vi "Read_Bid.vi"(8 "error in (no error)":errorcluster, 11 "Modbus master in":refnum<class "Modbus Master.lvclass">) -> (0 "error out":errorcluster, 2 "Variables":sgl[](array[numeric]), 3 "Modbus master out":refnum<class "Modbus Master.lvclass">)   [LabVIEW 2017]
uses:
  <vilib>/Modbus/master/Modbus Master.lvclass
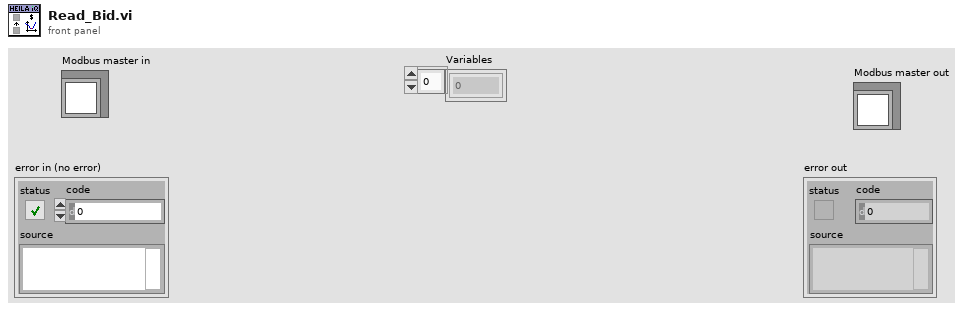
[diagram p1: front panel]
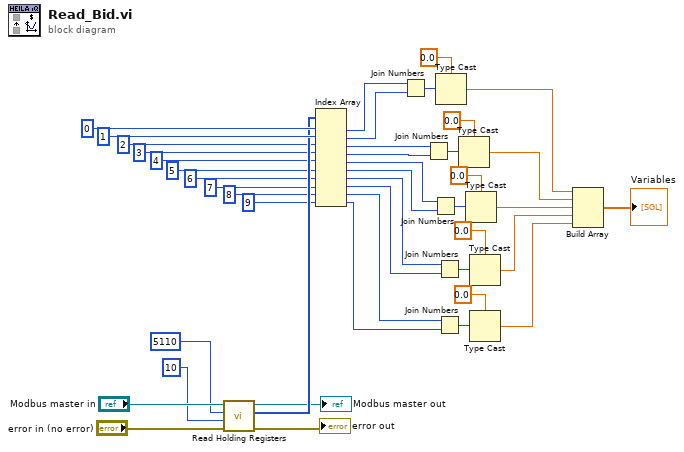
[diagram p0: block diagram]
diagram:
  n1 = call-dynamic "Read Holding Registers.vi"("error in (no error)"="error in (no error)", "number of holding registers"=u16 10 ("starting address"), "starting address"=u16 5110, "Modbus master in"="Modbus master in") -> ("error out"=→"error out":errorcluster, "register values"=w37:u16[], "Modbus master out"=→"Modbus master out":refnum<class "Modbus Master.lvclass">)  [unwired: 5 in]
  n2 = Index Array(array=w37, index #1=0 ("index"), index #2=1 ("index"), index #3=2 ("index"), index #4=3 ("index"), index #5=4 ("index"), index #6=5 ("index"), index #7=6 ("index"), index #8=7 ("index"), index #9=8 ("index"), index #10=9 ("index")) -> (element #1=w33:u16, element #2=w34:u16, element #3=w18:u16, element #4=w17:u16, element #5=w13:u16, element #6=w12:u16, element #7=w7:u16, element #8=w6:u16, element #9=w5:u16, element #10=w4:u16)
  n3 = Join Numbers(hi=w33, lo=w34) -> ((hi.lo)=w32:u32)
  n4 = Join Numbers(hi=w18, lo=w17) -> ((hi.lo)=w20:u32)
  n5 = Join Numbers(hi=w13, lo=w12) -> ((hi.lo)=w15:u32)
  n6 = Join Numbers(hi=w7, lo=w6) -> ((hi.lo)=w11:u32)
  n7 = Join Numbers(hi=w5, lo=w4) -> ((hi.lo)=w9:u32)
  n8 = Type Cast(type=sgl 0.0, x=w32) -> (*(type *) &x=w30:sgl)
  n9 = Type Cast(type=sgl 0.0, x=w20) -> (*(type *) &x=w16:sgl)
  n10 = Type Cast(type=sgl 0.0, x=w15) -> (*(type *) &x=w3:sgl)
  n11 = Type Cast(type=sgl 0.0, x=w11) -> (*(type *) &x=w2:sgl)
  n12 = Type Cast(type=sgl 0.0, x=w9) -> (*(type *) &x=w1:sgl)
  n13 = Build Array(w30, w16, w3, w2, w1) -> (→"Variables":sgl[])
